vi "LightState(SubVI).vi"(5 "Button number(1-5)":dbl, 6 "Red":refnum<vi>, 7 "State":enum16{"Wrong", "Stopped", "Right"}(ring), 8 "White":refnum<vi>, 9 "Blue":refnum<vi>, 10 "Yellow":refnum<vi>, 11 "Green":refnum<vi>) -> (0 "Button 4":bool, 1 "Button 3":bool, 2 "Button 2":bool, 3 "Button1":bool, 4 "Button 5":bool)   [LabVIEW 2014]
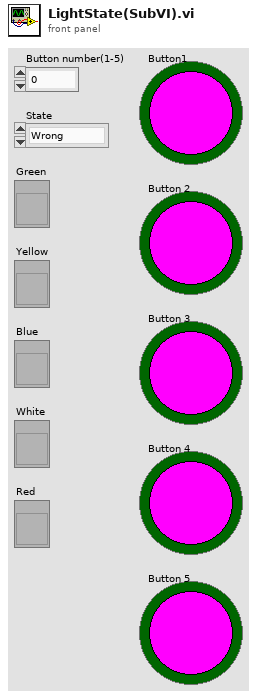
[diagram p1: front panel]
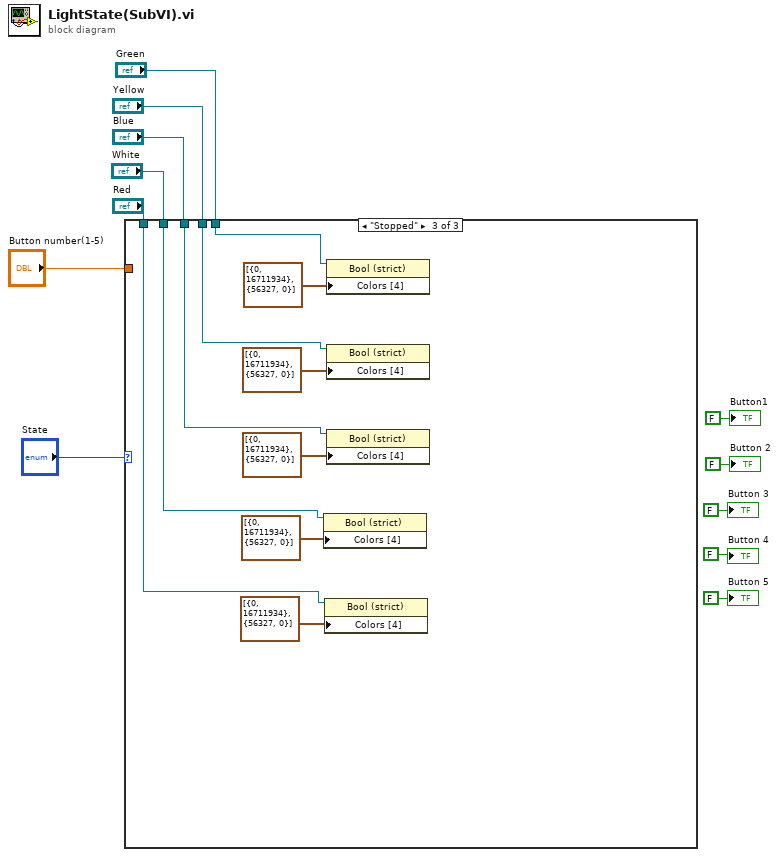
[diagram p0: block diagram]
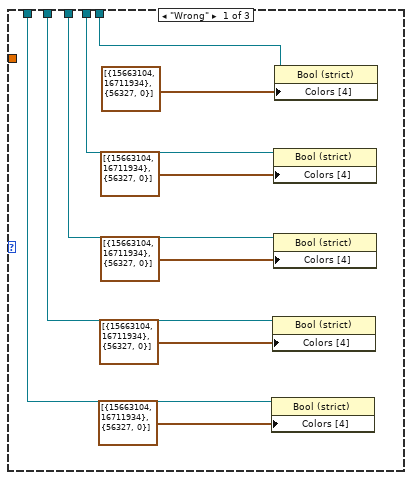
[diagram p2: hidden frame]
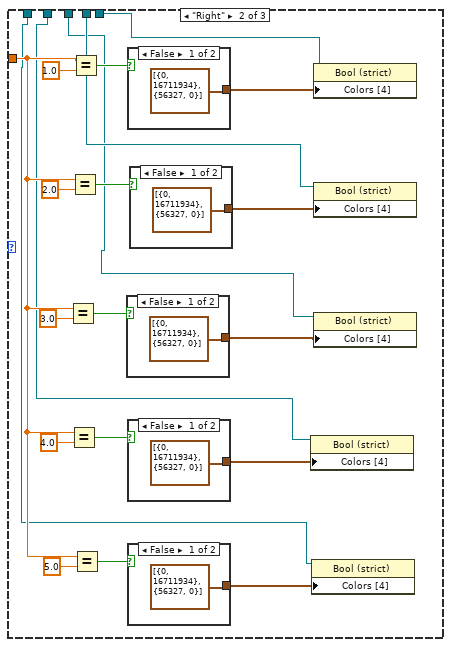
[diagram p3: hidden frame]
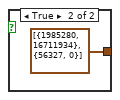
[diagram p4: hidden frame]
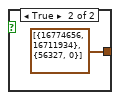
[diagram p5: hidden frame]
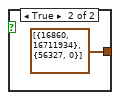
[diagram p6: hidden frame]
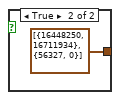
[diagram p7: hidden frame]
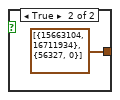
[diagram p8: hidden frame]
diagram:
  n1 = case shown="\"Stopped\"" "State" {
    tunnel: "Button number(1-5)" -> [_ w28 _]
    tunnel: "Green" -> [w17 w27 w58]
    tunnel: "Yellow" -> [w16 w26 w57]
    tunnel: "Blue" -> [w15 w25 w56]
    tunnel: "White" -> [w14 w24 w55]
    tunnel: "Red" -> [w13 w23 w54]
    frame "Wrong" {
      n2 = property on="Property Node" class="Bool (strict)"(reference=w13, "Colors [4]"=cluster{u32, u32}[] [{15663104, 16711934}, {56327, 0}]) -> ()  [unwired: 1 in, 2 out]
      n3 = property on="Property Node" class="Bool (strict)"(reference=w14, "Colors [4]"=cluster{u32, u32}[] [{15663104, 16711934}, {56327, 0}]) -> ()  [unwired: 1 in, 2 out]
      n4 = property on="Property Node" class="Bool (strict)"(reference=w16, "Colors [4]"=cluster{u32, u32}[] [{15663104, 16711934}, {56327, 0}]) -> ()  [unwired: 1 in, 2 out]
      n5 = property on="Property Node" class="Bool (strict)"(reference=w15, "Colors [4]"=cluster{u32, u32}[] [{15663104, 16711934}, {56327, 0}]) -> ()  [unwired: 1 in, 2 out]
      n6 = property on="Property Node" class="Bool (strict)"(reference=w17, "Colors [4]"=cluster{u32, u32}[] [{15663104, 16711934}, {56327, 0}]) -> ()  [unwired: 1 in, 2 out]
    }
    frame "Right" {
      n7 = Equal?(x=w28, y=3.0) -> (x = y?=w35:bool)
      n8 = Equal?(x=w28, y=4.0) -> (x = y?=w36:bool)
      n9 = Equal?(x=w28, y=2.0) -> (x = y?=w34:bool)
      n10 = Equal?(x=w28, y=1.0) -> (x = y?=w38:bool)
      n11 = Equal?(x=w28, y=5.0) -> (x = y?=w37:bool)
      n12 = case shown="False" w35 {
        tunnel: [cluster{u32, u32}[] [{0, 16711934}, {56327, 0}] cluster{u32, u32}[] [{16860, 16711934}, {56327, 0}]] -> w41
        frame False {
        }
        frame True {
        }
      }
      n13 = case shown="False" w38 {
        tunnel: [cluster{u32, u32}[] [{0, 16711934}, {56327, 0}] cluster{u32, u32}[] [{1985280, 16711934}, {56327, 0}]] -> w39
        frame False {
        }
        frame True {
        }
      }
      n14 = case shown="False" w36 {
        tunnel: [cluster{u32, u32}[] [{0, 16711934}, {56327, 0}] cluster{u32, u32}[] [{16448250, 16711934}, {56327, 0}]] -> w42
        frame False {
        }
        frame True {
        }
      }
      n15 = case shown="False" w37 {
        tunnel: [cluster{u32, u32}[] [{0, 16711934}, {56327, 0}] cluster{u32, u32}[] [{15663104, 16711934}, {56327, 0}]] -> w43
        frame False {
        }
        frame True {
        }
      }
      n16 = case shown="False" w34 {
        tunnel: [cluster{u32, u32}[] [{0, 16711934}, {56327, 0}] cluster{u32, u32}[] [{16774656, 16711934}, {56327, 0}]] -> w40
        frame False {
        }
        frame True {
        }
      }
      n17 = property on="Property Node" class="Bool (strict)"(reference=w24, "Colors [4]"=w42) -> ()  [unwired: 1 in, 2 out]
      n18 = property on="Property Node" class="Bool (strict)"(reference=w23, "Colors [4]"=w43) -> ()  [unwired: 1 in, 2 out]
      n19 = property on="Property Node" class="Bool (strict)"(reference=w27, "Colors [4]"=w39) -> ()  [unwired: 1 in, 2 out]
      n20 = property on="Property Node" class="Bool (strict)"(reference=w26, "Colors [4]"=w40) -> ()  [unwired: 1 in, 2 out]
      n21 = property on="Property Node" class="Bool (strict)"(reference=w25, "Colors [4]"=w41) -> ()  [unwired: 1 in, 2 out]
    }
    frame "Stopped" {
      n22 = property on="Property Node" class="Bool (strict)"(reference=w55, "Colors [4]"=cluster{u32, u32}[] [{0, 16711934}, {56327, 0}]) -> ()  [unwired: 1 in, 2 out]
      n23 = property on="Property Node" class="Bool (strict)"(reference=w54, "Colors [4]"=cluster{u32, u32}[] [{0, 16711934}, {56327, 0}]) -> ()  [unwired: 1 in, 2 out]
      n24 = property on="Property Node" class="Bool (strict)"(reference=w58, "Colors [4]"=cluster{u32, u32}[] [{0, 16711934}, {56327, 0}]) -> ()  [unwired: 1 in, 2 out]
      n25 = property on="Property Node" class="Bool (strict)"(reference=w57, "Colors [4]"=cluster{u32, u32}[] [{0, 16711934}, {56327, 0}]) -> ()  [unwired: 1 in, 2 out]
      n26 = property on="Property Node" class="Bool (strict)"(reference=w56, "Colors [4]"=cluster{u32, u32}[] [{0, 16711934}, {56327, 0}]) -> ()  [unwired: 1 in, 2 out]
    }
  }
  "Button1" <- FALSE ("Button1")
  "Button 2" <- FALSE ("Button 2")
  "Button 3" <- FALSE ("Button 3")
  "Button 4" <- FALSE ("Button 4")
  "Button 5" <- FALSE ("Button 5")
